vi "Pop Up Channel Data.vi"(11 "Channels in":T1 {"Mapping"."VS Reference" format="%.0x"}) -> ()   [LabVIEW 2021, in "Modbus Master System Explorer.lvlib"]
uses:
  Modbus Master System Explorer.lvlib
  Shared/Controls/Data Model/Channel.ctl
  SubVIs/Modbus Type.ctl
  <vilib>/NI VeriStand/Custom Device API/Custom Device Channel Type.ctl
  Shared/Controls/Data Model/Mapping.ctl
  Shared/Controls/Data Model/DataType.ctl
  <vilib>/NI VeriStand/Custom Device API/Custom Device Item Ref.ctl
  Shared/Modbus Master Shared.lvlib
  <vilib>/NI VeriStand/Custom Device API/Custom Device API.lvlib
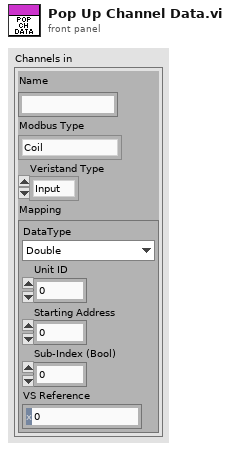
[diagram p1: front panel]
types:
  T1 = typedef "Modbus Master Shared.lvlib/Channel.ctl" = cluster{"Name":string, "Modbus Type":T2, "Veristand Type":T3, "Mapping":T4}
  T2 = typedef "Modbus Master Shared.lvlib/Modbus Type.ctl" = enum16{"Coil", "Discrete Input", "Holding Register", "Input Register"}
  T3 = typedef "Custom Device API.lvlib/Custom Device Channel Type.ctl" = enum16{"Input", "Output"}
  T4 = typedef "Modbus Master Shared.lvlib/Mapping.ctl" = cluster{"DataType":T5, "Unit ID":u8, "Starting Address":u16, "Sub-Index (Bool)":u16, "VS Reference":T6}
  T5 = typedef "Modbus Master Shared.lvlib/DataType.ctl" = enum16{"Double", "Single", "I64", "I32", "I16", "I8", "U64", "U32", "U16", "U8", "Boolean"}
  T6 = typedef "Custom Device API.lvlib/Custom Device Item Ref.ctl" = u64
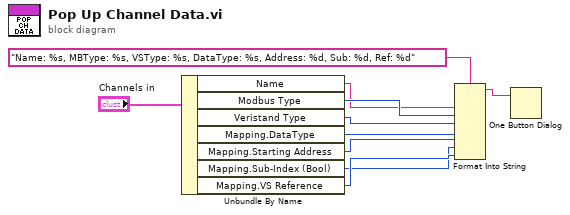
[diagram p0: block diagram]
diagram:
  n1 = Unbundle By Name("Channels in") -> ("Name"=w3:string, "Modbus Type"=w4:T2, "Veristand Type"=w5:T3, "Mapping.DataType"=w6:T5, "Mapping.Starting Address"=w7:u16, "Mapping.Sub-Index (Bool)"=w8:u16, "Mapping.VS Reference"=w9:T6)
  n2 = Format Into String(format string="Name: %s, MBType: %s, VSType: %s, DataType: %s, Address: %d, Sub: %d, Ref: %d", w3, w4, w5, w6, w7, w8, w9) -> (resulting string=w10:string)  [unwired: 2 in, 1 out]
  n3 = One Button Dialog(message=w10) -> ()  [unwired: 1 in, 1 out]
